vi "Create Numeric Control.vi"(4 "Terminal Position":T1, 5 "Sink/Source":refnum<vi>, 6 "FP Position":T1, 8 "error in (no error)":errorcluster, 9 "Indicator":bool, 10 "Value":variant, 11 "Diagram":refnum<vi>) -> (0 "error out":errorcluster, 2 "Output Terminal":refnum<vi>, 3 "Control Ref":refnum<vi>)   [LabVIEW 2018, in "Scripting Tools.lvlib"]
uses:
  Scripting Tools.lvlib
  <vilib>/Utility/miscctls.llb/LVPointTypeDef.ctl
  <vilib>/Utility/VariantDataType/VariantType.lvlib
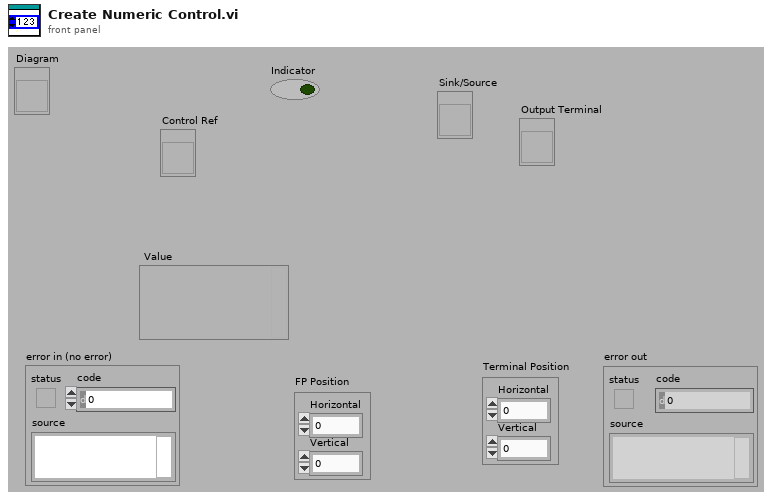
[diagram p1: front panel]
types:
  T1 = typedef "LVPointTypeDef.ctl" = cluster{"Horizontal":i16, "Vertical":i16}
  T2 = typedef "VariantType.lvlib/Type.ctl" = enum8{"Invalid Type", "Void", "I8", "I16", "I32", "I64", "U8", "U16", "U32", "U64", "Single Float", "Double Float", "Extended Float", "Single Complex", "Double Complex", "Extended Complex", "Enum U8", "Enum U16", "Enum U32", "Enum U64", "Single Float With Unit", "Double Float With Unit", "Extended Float With Unit", "Single Complex with Unit", "Double Complex with Unit", "Extended Complex with Unit", "Boolean", "String", "Path", "Picture", "Tag", "Array", "Cluster", "Variant", "LV Variant", "Waveform", "Timestamp", "Digital Waveform", "Digital Data", "ExpressData", "Refnum", "External Data", "VI", "Poly VI", "LabVIEW Class Instance", "Fixed Point"}
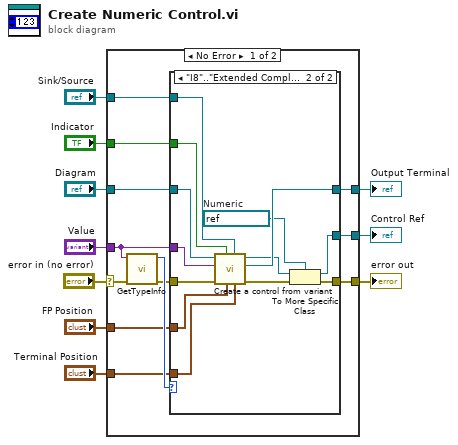
[diagram p0: block diagram]
diagram:
  n1 = case shown="No Error" "error in (no error)" {
    selector: "error in (no error)" -> [w22 w37]
    tunnel: [w14 w37] -> w10
    tunnel: "Diagram" -> [w19 _]
    tunnel: "Value" -> [w18 _]
    tunnel: "FP Position" -> [w17 _]
    tunnel: [w16 _] -> w5
    tunnel: [w15 _] -> w4
    tunnel: "Sink/Source" -> [w13 _]
    tunnel: "Indicator" -> [w12 _]
    tunnel: "Terminal Position" -> [w11 _]
    frame No Error {
      n2 = call <vilib>:"GetTypeInfo.vi"("error in (no error)"=w22, "Variant"=w18) -> ("error out"=w20:errorcluster, "Type Enum"=w21:T2)  [unwired: 8 out]
      n3 = case shown="\"I8\"..\"Extended Complex with Unit\"" w21 {
        tunnel: w20 -> [w23 w34]
        tunnel: w19 -> [_ w36]
        tunnel: w18 -> [_ w35]
        tunnel: w17 -> [_ w33]
        tunnel: [_ w31] -> w16
        tunnel: [_ w29] -> w15
        tunnel: [w23 w28] -> w14
        tunnel: w13 -> [_ w27]
        tunnel: w12 -> [_ w26]
        tunnel: w11 -> [_ w24]
        frame "Invalid Type", Default {
        }
        frame "I8".."Extended Complex with Unit" {
          w30 = refnum<vi> refnum  # Numeric
          n4 = call "Create a control from variant.vi"("Terminal Position"=w24, "Terminal Source/Sink"=w27, "FP position"=w33, "Indicator?"=w26, "error in (no error)"=w34, "Constant Data"=w35, "Diagram"=w36) -> ("error out"=w32:errorcluster, "Terminal"=w31:refnum<vi>, "Control Reference"=w25:refnum<vi>)  [unwired: 2 out]
          n5 = To More Specific Class(target class=w30, reference=w25, error in=w32) -> (specific class reference=w29:refnum<vi>, error out=w28:errorcluster)
        }
      }
    }
    frame Error {
    }
  }
  "error out" <- w10
  "Output Terminal" <- w5
  "Control Ref" <- w4
